vi "SDCP SMF Receiver and Transmitter - Test.vi"() -> ()   [LabVIEW 2020]
uses:
  Typedefs/SDCP - Serial Port Control - Commands.ctl
  Typedefs/SDCP - Standard Message Frame Parameters - FGV - commands.ctl
  <vilib>/Utility/miscctls.llb/LVComboBoxStrsAndValuesArrayTypeDef.ctl
  Global Stop.vi
panel:
  in  "Stop recording at time":bool
  in  "Stop time (ms)":u32
  in  "Synchronize":bool
  in  "Number of frames \nto request":u8
  in  "Request frames":bool
  in  "Frame IDs to request":u8[](array[numeric])=[0, 0, 0, 0, 0, 0, 0]
  in  "Remove frame":bool
  in  "Frame to add":string(combo)
  in  "Add frame":bool
  in  "Transmit Table":string[][](table)
  out "Elapsed time (ms)":u32
  in  "Parameter file path":path=path "E:/Projects/System Diagnostics and Control Protocol/SDCP_LabVIEW/Parameter Files/Motion_Processing.param"
  in  "Receive Table":i32(listbox)
  in  "stop":bool
  in  "VISA resource name":refnum<visa-resource-name>
  in  "Baud rate":u32=9600
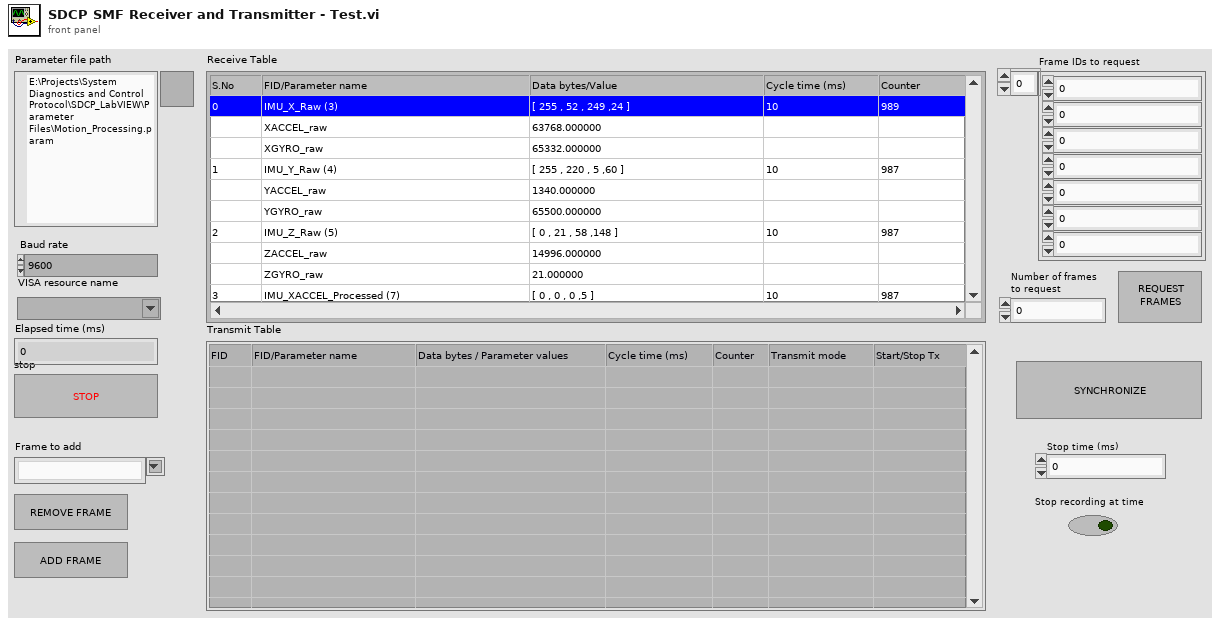
[diagram p1: front panel]
types:
  T1 = enum16{"Initialize", "Add row", "Remove row", "Update"}
  T2 = typedef "LVComboBoxStrsAndValuesArrayTypeDef.ctl" = cluster{"String":string, "Value":string}[]
  T3 = typedef "SDCP - Standard Message Frame Parameters - FGV - commands.ctl" = enum16{"Write descriptors", "Read descriptors", "Read values", "Load parameters from file", "Write values", "Read all descriptors"}
  T4 = typedef "SDCP - Serial Port Control - Commands.ctl" = enum16{"Open", "Read", "Write", "Get instance", "Close"}
  T5 = typedef "SDCP - SMF parameter descriptors.ctl" = cluster{"Frame name":string, "Frame ID":i32, "Data type":string, "Start Position":i32, "Length":i32, "Factor":dbl, "Offset":dbl, "Parameter name":string, "Value":string}
  T6 = typedef "SDCP SMF Receiver and Transmitter - Notifier and Queues.ctl" = cluster{"Trace Queue":refnum<queue>, "Tx - Log Table Queue":refnum<queue>, "Tx - User Queue":refnum<queue>, "Rx - Log Table Queue":refnum<queue>, "Rx - User Queue":refnum<queue>, "Log status Notifier":refnum<notifier>, "Plot Queue":refnum<queue>}
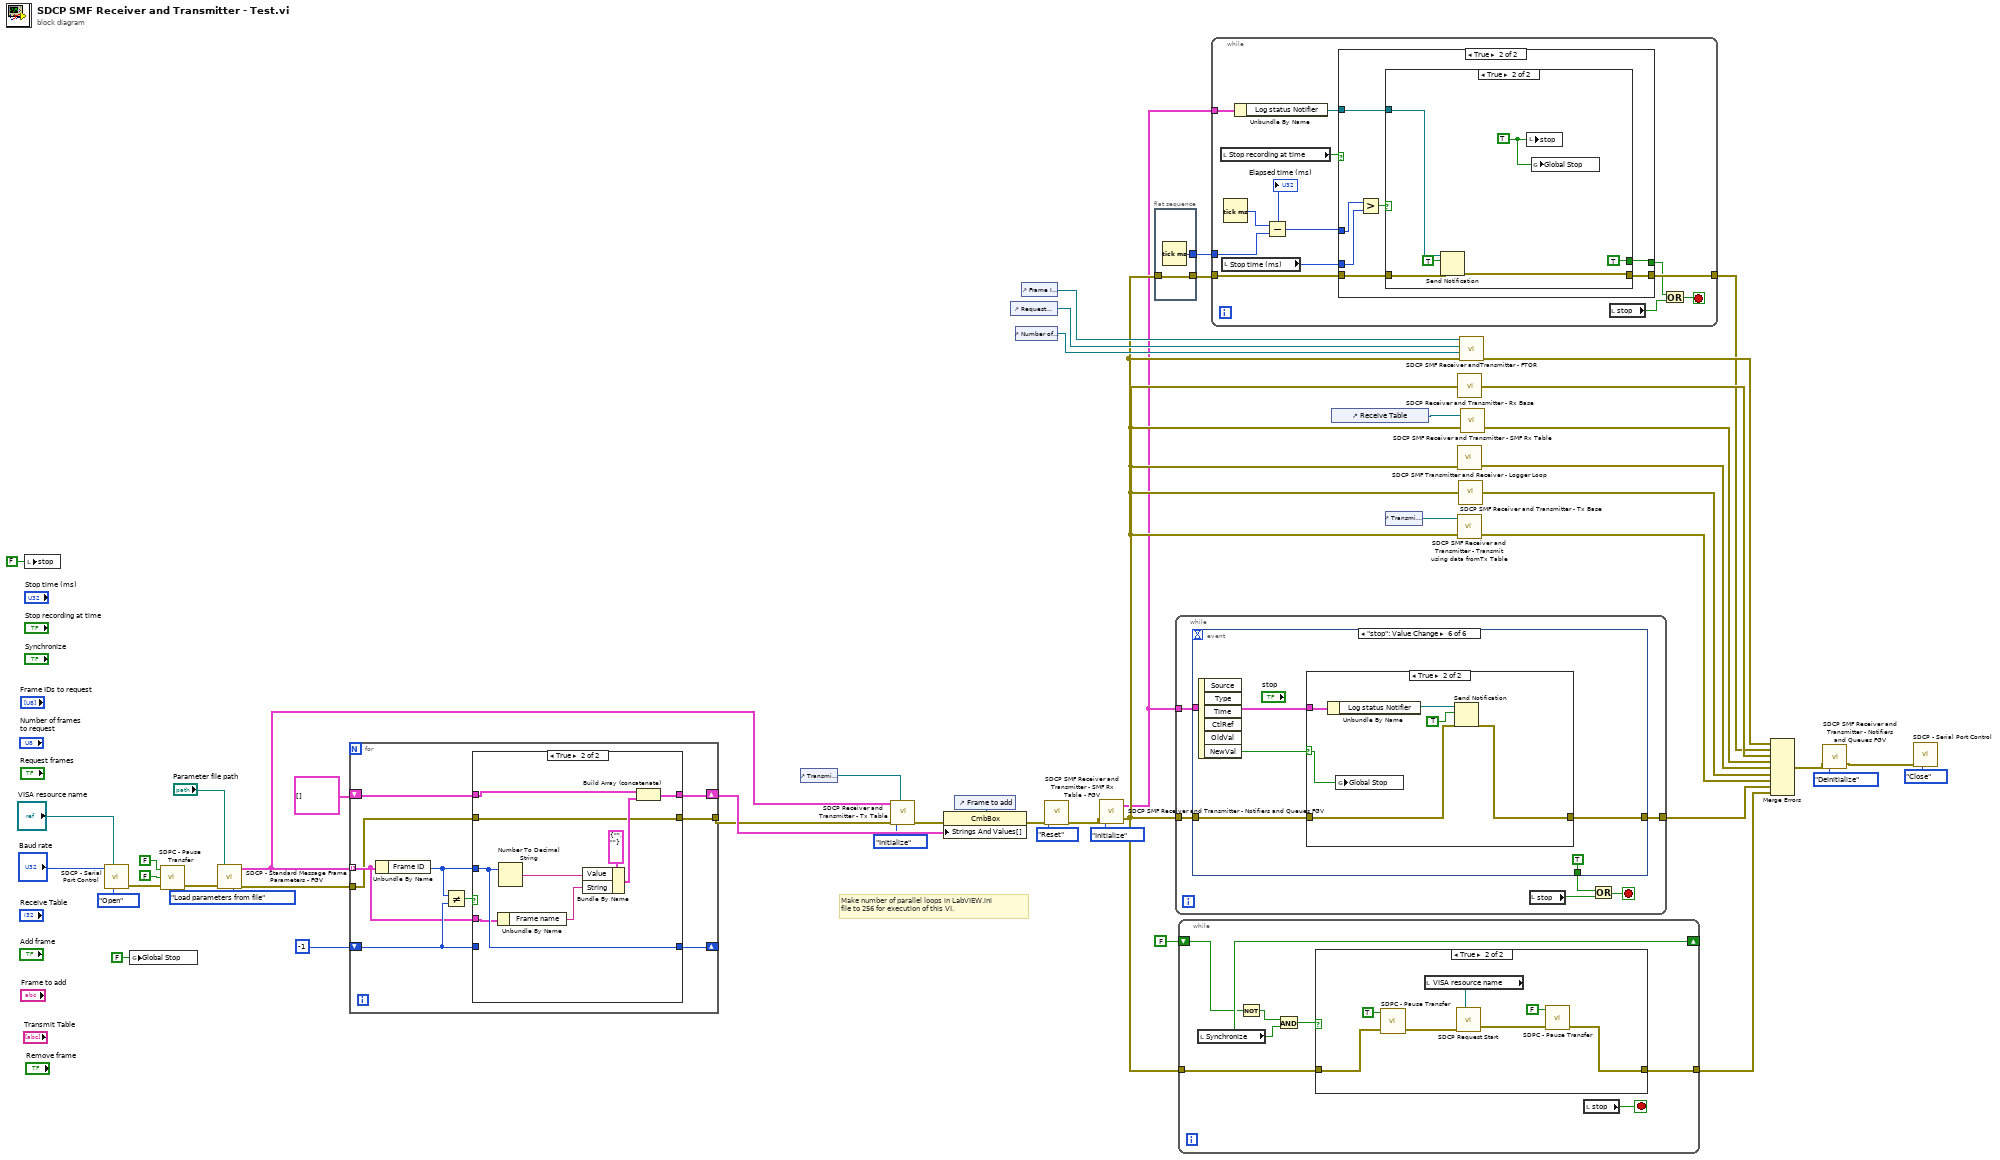
[diagram p0: block diagram]
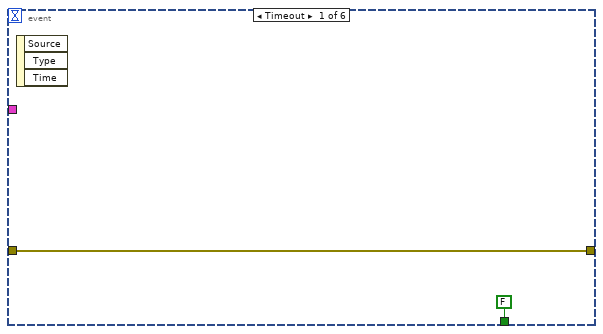
[diagram p3: hidden frame]
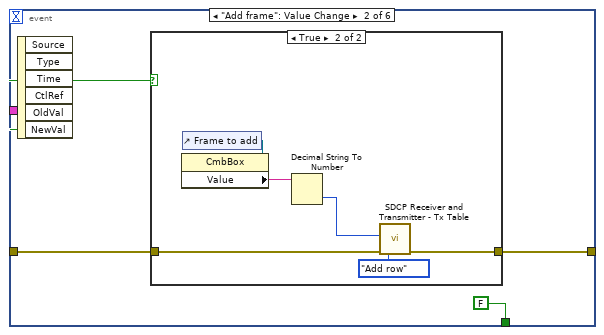
[diagram p4: hidden frame]
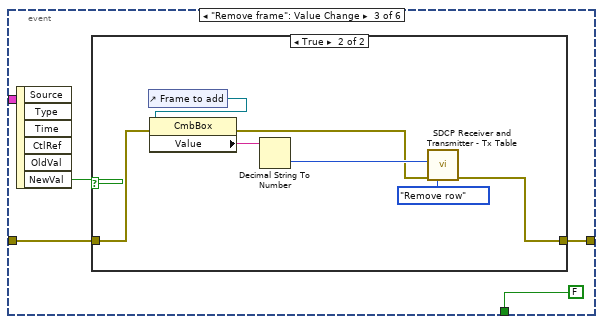
[diagram p6: hidden frame]
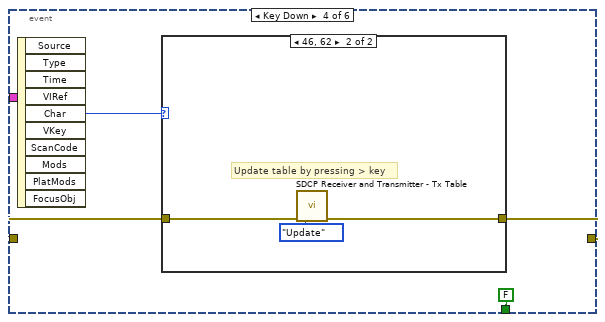
[diagram p8: hidden frame]
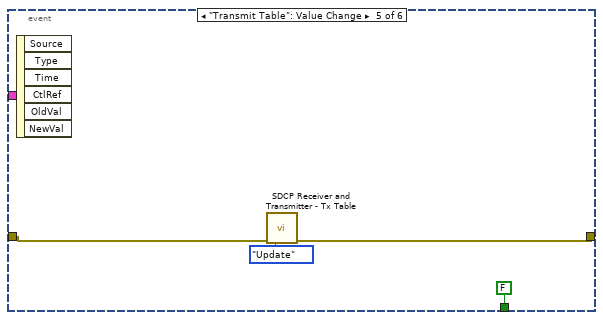
[diagram p10: hidden frame]
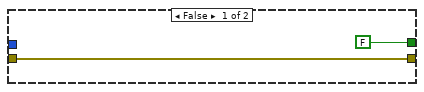
[diagram p13: hidden frame]
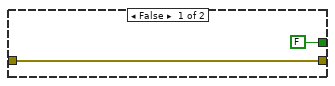
[diagram p14: hidden frame]
diagram:
  # "Make number of parallel loops in LabVIEW.ini\nfile to 256 for execution of this VI."
  n1 = local write "stop"(FALSE ("stop")) -> ()
  n2 = call "SDCP - Serial Port Control.vi"("Command"=SDCP_-_Serial_Port_Control_-_Commands."Open", "VISA resource name"="VISA resource name", "Baud rate"="Baud rate") -> ("error out"=w18:errorcluster)  [unwired: 5 in, 3 out]
  n3 = global write "Global Stop.vi" "Global Stop"(FALSE ("Global Stop")) -> ()
  n4 = call "SDPC - Pause Transfer.vi"("error in (no error)"=w18, "RD/nWR"=FALSE, "Pause transfer"=FALSE) -> ("error out"=w17:errorcluster)  [unwired: 1 in, 1 out]
  n5 = call "SDCP - Standard Message Frame Parameters - FGV.vi"("Parameter file path"="Parameter file path", "error in (no error)"=w17, "Command"=SDCP_-_Standard_Message_Frame_Parameters_-_FGV_-_commands."Load parameters from file") -> ("SMF Parameters descriptors out"=w28:T5[], "error out"=w34:errorcluster)  [unwired: 4 in]
  n6 = for {
    tunnel: w34 -> [w50]
    tunnel: w28 -> [w51] mode=indexing
    shift-right: [w55] -> _
    shift-left: -1 -> [w54]
    shift-right: [w52] -> w30
    shift-left: T2 [] ("Strings And Values []") -> [w53]
    tunnel: [w49] -> w29
    n7 = Unbundle By Name(w51) -> ("Frame ID"=w56:i32)
    n8 = Not Equal?(x=w56, y=w54) -> (x != y?=w57:bool)
    n9 = case shown="True" w57 {
      tunnel: w56 -> [_ w69]
      tunnel: [w60 w69] -> w55
      tunnel: w54 -> [w60 _]
      tunnel: w53 -> [w59 w64]
      tunnel: [w59 w62] -> w52
      tunnel: w51 -> [_ w66]
      tunnel: w50 -> [w58 w61]
      tunnel: [w58 w61] -> w49
      frame False {
      }
      frame True {
        n10 = Unbundle By Name(w66) -> ("Frame name"=w65:string)
        n11 = Number To Decimal String(number=w69) -> (decimal integer string=w67:string)  [unwired: 1 in]
        n12 = Bundle By Name(cluster=cluster{"String":string, "Value":string} {"String"="", "Value"=""}, "Value"=w67, "String"=w65) -> (w63:cluster{"String":string, "Value":string})
        n13 = Build Array (concatenate)(w64, w63) -> (w62:T2)
      }
    }
  }
  n14 = control-ref of="Transmit Table"() -> (w25:refnum<vi>)
  n15 = call "SDCP Receiver and Transmitter - Tx Table.vi"("Table Control"=w25, "error in (no error)"=w29, "Command"=T1."Initialize", "SMF Parameters descriptors"=w28) -> ("error out"=w23:errorcluster)  [unwired: 6 in, 1 out]
  n16 = control-ref of="Frame to add"() -> (w24:refnum<vi>)
  n17 = property class="CmbBox"(reference=w24, error in=w23, "Strings And Values[]"=w30) -> (error out=w31:errorcluster)  [unwired: 1 out]
  n18 = control-ref of="Request frames"() -> (w11:refnum<vi>)
  n19 = control-ref of="Number of frames \nto request"() -> (w10:refnum<vi>)
  n20 = control-ref of="Frame IDs to request"() -> (w12:refnum<vi>)
  n21 = call "SDCP SMF Receiver and Transmitter - SMF Rx Table - FGV.vi"("error in (no error)"=w31, "Command"=enum16{"Reset", "Write", "Read"}."Reset") -> ("error out"=w41:errorcluster)  [unwired: 8 in, 1 out]
  n22 = call "SDCP SMF Receiver and Transmitter - Notifiers and Queues FGV.vi"("error in (no error)"=w41, "Command"=enum16{"Initialize", "Read", "Deinitialize"}."Initialize") -> ("error out"=w3:errorcluster, "Output"=w2:T6)
  n23 = flat-sequence {
    tunnel: [w71] -> w35
    tunnel: [w70] -> w7
    tunnel: w3 -> [w70]
    frame #0 {
      n24 = Tick Count (ms)() -> (millisecond timer value=w71:u32)
    }
  }
  n25 = while {
    tunnel: w3 -> [w77]
    tunnel: [w76] -> w19
    tunnel: w2 -> [w75]
    stop <- w74 stop-if-true
    n26 = event shown="[5] \"stop\": Value Change" {
      selector: _ -> [_ _ _ _ _ _]
      dyn-events: _ -> [_ _ _ _ _ _]
      timeout: _ -> [_ _ _ _ _ _]
      tunnel: w77 -> [w79 w82 w94 w105 w113 w116]
      tunnel: [w79 w81 w93 w104 w112 w115] -> w76
      tunnel: [FALSE FALSE FALSE FALSE FALSE TRUE] -> w73
      tunnel: w75 -> [_ _ _ _ _ w118]
      event Timeout {
        n27 = event-data() -> ()  [unwired: 1 in, 3 out]
      }
      event "Add frame": Value Change {
        n28 = event-data() -> ("NewVal"=w83:bool)  [unwired: 1 in, 5 out]
        n29 = case shown="True" w83 {
          tunnel: w82 -> [w84 w88]
          tunnel: [w84 w86] -> w81
          frame False {
          }
          frame True {
            n30 = control-ref of="Frame to add"() -> (w90:refnum<vi>)
            n31 = property class="CmbBox"(reference=w90) -> ("Value"=w89:string)  [unwired: 1 in, 2 out]
            n32 = Decimal String To Number(string=w89) -> (number=w87:i32)  [unwired: 2 in, 1 out]
            n33 = call "SDCP Receiver and Transmitter - Tx Table.vi"("error in (no error)"=w88, "Command"=T1."Add row", "FID"=w87) -> ("error out"=w86:errorcluster)  [unwired: 7 in, 1 out]
          }
        }
      }
      event "Remove frame": Value Change {
        n34 = event-data() -> ("NewVal"=w92:bool)  [unwired: 1 in, 5 out]
        n35 = case shown="True" w92 {
          tunnel: w94 -> [w95 w100]
          tunnel: [w95 w97] -> w93
          frame False {
          }
          frame True {
            n36 = control-ref of="Frame to add"() -> (w99:refnum<vi>)
            n37 = property class="CmbBox"(reference=w99, error in=w100) -> (error out=w98:errorcluster, "Value"=w102:string)  [unwired: 1 out]
            n38 = Decimal String To Number(string=w102) -> (number=w101:i32)  [unwired: 2 in, 1 out]
            n39 = call "SDCP Receiver and Transmitter - Tx Table.vi"("error in (no error)"=w98, "Command"=T1."Remove row", "FID"=w101) -> ("error out"=w97:errorcluster)  [unwired: 7 in, 1 out]
          }
        }
      }
      event Key Down {
        n40 = event-data() -> ("Char"=w103:i16)  [unwired: 1 in, 9 out]
        n41 = case shown="46, 62" w103 {
          tunnel: w105 -> [w107 w109]
          tunnel: [w107 w108] -> w104
          frame 0, Default {
          }
          frame 46, 62 {
            # "Update table by pressing > key"
            n42 = call "SDCP Receiver and Transmitter - Tx Table.vi"("error in (no error)"=w109, "Command"=T1."Update") -> ("error out"=w108:errorcluster)  [unwired: 8 in, 1 out]
          }
        }
      }
      event "Transmit Table": Value Change {
        n43 = event-data() -> ()  [unwired: 1 in, 6 out]
        n44 = call "SDCP Receiver and Transmitter - Tx Table.vi"("error in (no error)"=w113, "Command"=T1."Update") -> ("error out"=w112:errorcluster)  [unwired: 8 in, 1 out]
      }
      event "stop": Value Change {
        n45 = event-data() -> ("NewVal"=w117:bool)  [unwired: 1 in, 5 out]
        n46 = case shown="True" w117 {
          selector: w117 -> [_ w121]
          tunnel: w118 -> [_ w126]
          tunnel: w116 -> [w120 w123]
          tunnel: [w120 w122] -> w115
          frame False {
          }
          frame True {
            n47 = Unbundle By Name(w126) -> ("Log status Notifier"=w125:refnum<notifier>)
            n48 = global write "Global Stop.vi" "Global Stop"(w121) -> ()
            n49 = Send Notification(notification=TRUE, notifier=w125, error in (no error)=w123) -> (error out=w122:errorcluster)  [unwired: 1 out]
          }
        }
      }
    }
    n50 = local read "stop"() -> (w72:bool)
    n51 = Or(x=w73, y=w72) -> (x .or. y?=w74:bool)
  }
  n52 = while {
    tunnel: w3 -> [w128]
    shift-right: [w133] -> _
    shift-left: FALSE -> [w131]
    tunnel: [w127] -> w8
    stop <- w130 stop-if-true
    n53 = local read "Synchronize"() -> (w133:bool)
    n54 = Not(x=w131) -> (.not. x?=w132:bool)
    n55 = And(x=w132, y=w133) -> (x .and. y?=w129:bool)
    n56 = case shown="True" w129 {
      tunnel: w128 -> [w134 w140]
      tunnel: [w134 w135] -> w127
      frame False {
      }
      frame True {
        n57 = call "SDPC - Pause Transfer.vi"("error in (no error)"=w140, "Pause transfer"=TRUE) -> ("error out"=w138:errorcluster)  [unwired: 2 in, 1 out]
        n58 = local read "VISA resource name"() -> (w141:refnum<visa-resource-name>)
        n59 = call "SDCP Request Start.vi"("error in (no error)"=w138, "COM Port"=w141) -> ("error out"=w137:errorcluster)  [unwired: 1 out]
        n60 = call "SDPC - Pause Transfer.vi"("error in (no error)"=w137, "Pause transfer"=FALSE) -> ("error out"=w135:errorcluster)  [unwired: 2 in, 1 out]
      }
    }
    n61 = local read "stop"() -> (w130:bool)
  }
  n62 = while {
    tunnel: w7 -> [w149]
    tunnel: w35 -> [w152]
    tunnel: [w148] -> w6
    tunnel: w2 -> [w143]
    stop <- w151 stop-if-true
    n63 = local read "Stop recording at time"() -> (w147:bool)
    n64 = local read "Stop time (ms)"() -> (w144:u32)
    n65 = Tick Count (ms)() -> (millisecond timer value=w153:u32)
    n66 = Unbundle By Name(w143) -> ("Log status Notifier"=w142:refnum<notifier>)
    n67 = Subtract(x=w153, y=w152) -> (x-y=w146:u32)
    "Elapsed time (ms)" <- w146
    n68 = case shown="True" w147 {
      tunnel: w149 -> [w155 w160]
      tunnel: [w155 w158] -> w148
      tunnel: w146 -> [_ w162]
      tunnel: [FALSE w157] -> w145
      tunnel: w144 -> [_ w161]
      tunnel: w142 -> [_ w156]
      frame False {
      }
      frame True {
        n69 = Greater?(x=w162, y=w161) -> (0:w159:bool)
        n70 = case shown="True" w159 {
          tunnel: w160 -> [w163 w170]
          tunnel: [w163 w167] -> w158
          tunnel: [FALSE TRUE] -> w157
          tunnel: w156 -> [_ w169]
          frame False {
          }
          frame True {
            w165 = TRUE ("stop")
            n71 = Send Notification(notification=TRUE, notifier=w169, error in (no error)=w170) -> (error out=w167:errorcluster)  [unwired: 1 out]
            n72 = local write "stop"(w165) -> ()
            n73 = global write "Global Stop.vi" "Global Stop"(w165) -> ()
          }
        }
      }
    }
    n74 = local read "stop"() -> (w150:bool)
    n75 = Or(x=w145, y=w150) -> (x .or. y?=w151:bool)
  }
  n76 = control-ref of="Receive Table"() -> (w39:refnum<vi>)
  n77 = control-ref of="Transmit Table"() -> (w22:refnum<vi>)
  n78 = call "SDCP SMF Transmitter and Receiver - Logger Loop.vi"("error in (no error)"=w3) -> ("error out"=w4:errorcluster)  [unwired: 3 in, 1 out]
  n79 = call "SDCP SMF Receiver and Transmitter - Transmit using data fromTx Table.vi"("error in (no error)"=w3, "Table Control"=w22) -> ("error out"=w20:errorcluster)  [unwired: 3 in]
  n80 = call "SDCP Receiver and Transmitter - Rx Base.vi"("error in (no error)"=w3) -> ("error out"=w14:errorcluster)
  n81 = call "SDCP SMF Receiver and Transmitter - Tx Base.vi"("error in (no error)"=w3) -> ("error out"=w21:errorcluster)
  n82 = call "SDCP SMF Receiver andTransmitter - FTOR.vi"("error in (no error)"=w3, "Number of requested frames"=w10, "Request frames"=w11, "FTOR FIDs"=w12) -> ("error out"=w13:errorcluster)  [unwired: 3 in]
  n83 = call "SDCP SMF Receiver and Transmitter - SMF Rx Table.vi"("error in (no error)"=w3, "Table reference"=w39) -> ("error out"=w38:errorcluster)  [unwired: 1 in]
  n84 = Merge Errors(w13, w6, w14, w38, w4, w21, w20, w19, w8) -> (w27:errorcluster)
  n85 = call "SDCP SMF Receiver and Transmitter - Notifiers and Queues FGV.vi"("error in (no error)"=w27, "Command"=enum16{"Initialize", "Read", "Deinitialize"}."Deinitialize") -> ("error out"=w43:errorcluster)  [unwired: 1 out]
  n86 = call "SDCP - Serial Port Control.vi"("Command"=SDCP_-_Serial_Port_Control_-_Commands."Close", "error in (no error)"=w43) -> ()  [unwired: 6 in, 4 out]
